vi "set_origin.vi"(2 "error in (no error)":errorcluster caption="错误输入（无错误）", 3 "value":i32, 4 "StepMotor输入":refnum<class "StepMotor.lvclass">) -> (0 "error out":errorcluster caption="错误输出", 1 "StepMotor输出":refnum<class "StepMotor.lvclass">)   [LabVIEW 2016, in "MotionControl.lvlib" / "StepMotor.lvclass"]
uses:
  <userlib>/MotionControl/StepMotor/StepMotor.lvclass
  <userlib>/MotionControl/StepMotor/StepMotor.lvclass/StepMotor.ctl
  <userlib>/UISimCanFunc_wrapper/UISimCanFunc_wrapper.lvlib
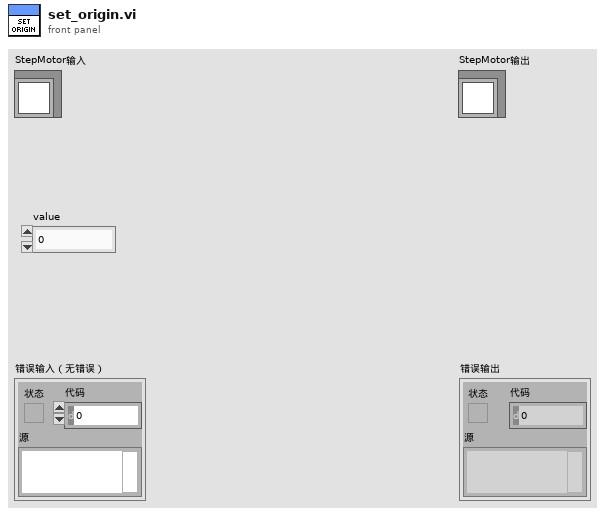
[diagram p1: front panel]
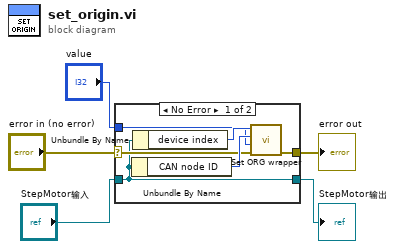
[diagram p0: block diagram]
diagram:
  n1 = case shown="No Error" "error in (no error)" {
    selector: "error in (no error)" -> [w8 w12]
    tunnel: [w7 w12] -> w4
    tunnel: [w6 w13] -> w2
    tunnel: "StepMotor输入" -> [w6 w13]
    tunnel: "value" -> [w9 _]
    frame No Error {
      n2 = Unbundle By Name(w6) -> ("CAN node ID"=w10:u32)
      n3 = Unbundle By Name(w6) -> ("device index"=w11:u32)
      n4 = call <userlib>:"Set ORG wrapper.vi"("error in (no error)"=w8, "iValue"=w9, "dwCanNodeId"=w10, "dwDevIndex"=w11) -> ("error out"=w7:errorcluster)  [unwired: 5 in, 2 out]
    }
    frame Error {
    }
  }
  "error out" <- w4
  "StepMotor输出" <- w2
